vi "UHR-Fleezers Control (host) - Lorentz v3.vi"() -> ()   [LabVIEW 2014] (continued)
  in  "Retract Pump 3":bool
  in  "Stop Flow":bool
  in  "Start Flow":bool
  in  "Flush Sample":bool
  in  "Volume (uL)":dbl=100.0
  in  "Flush rate (uL/m)":dbl=100.0
  in  "Flow rate (uL/h)":dbl=100.0
  in  "Clear Volume":bool caption="Clear Infused Volume"
  in  "Flush Pump 3":bool
  in  "Volume (uL) P3":dbl=150.0 caption="Volume (uL)"
  in  "Flush rate (uL/m) P3":dbl=100.0 caption="Rate (uL/m)"
  out "Flushing P1":bool caption="Flushing"
  in  "Volume (uL) P1":dbl=100.0 caption="Volume (uL)"
  in  "Flush rate (uL/m) P1":dbl=100.0 caption="Rate (uL/m)"
  in  "Normal Flow Rate (ul/h) P1":dbl=600.0 caption="Normal Flow Rate (ul/h)"
  in  "Flush Pump 1":bool
  in  "Clear Volume P3":bool caption="Clear Infused Volume"
  in  "Clear Volume P1":bool caption="Clear Infused Volume"
  in  "Display On P1":bool caption="Display On"
  in  "All Pump Parameters":T10={"Pump 1"={"Diameter (mm)"=4.61, "Units"=4.0, "Volume"=100.0, "Rate"=25.0}, "Pump 2"={"Diameter (mm)"=4.61, "Units"=3.0, "Volume"=0.0, "Rate"=0.0}, "Pump 3"={"Diameter (mm)"=4.61, "Units"=4.0, "Volume"=100.0, "Rate"=800.0}}
  in  "Total Volume\nFlushed (uL)":dbl
  in  "Inject Pump 2":bool caption="Inject Pump 2\n(Flush Center)"
  in  "Flush Center Ch Rate (ul/m)":dbl=100.0
  in  "Flush Center Ch Volume (uL)":dbl=15.0
  in  "Pump pause delay (ms)":u32
  in  "Pump write delay (ms)":dbl=300.0
  in  "Ch 3 Inject Rate (ul/h)":dbl=800.0
  in  "Ch 3 Inject Volume (uL)":dbl=100.0
  in  "Ch 1 Inject Volume (uL)":dbl=100.0
  in  "Ch 1 Inject Rate (ul/h)":dbl=25.0
  out "Pump 1 cont disp":string="Right: DNA beads "
  out "Pump 3 cont disp":string="Left: ADig beads"
  in  "Read Harvard":bool
  out "read buffer":string
  out "Serial Settings:Number of Bytes at Serial Port":u32
  in  "write buffer":string
  in  "Tab Control 2":T11(tab)=enum."Feedback on Trap Position"
  in  "Update all trap values":bool
  out "Total Counts (ticks)":u16=600
  in  "Trap ON/OFF X or Y Amp?":bool=TRUE
  in  "Oscillate Set 1":bool
  in  "Trap 1 ON":bool
  in  "Number Interlace Sets":u8=3 min=1 max=3
  in  "DIO count 3 (ticks)":u16=200
  in  "DIO count 2 (ticks)":u16=200
  in  "DIO count 1 (ticks)":u16=200
  in  "BD 2 Amplitude 3 (%)":dbl min=0.0 max=45.0 step=1.0
  in  "BD 2 Amplitude 2 (%)":dbl min=0.0 max=45.0 step=1.0
  in  "BD 2 Amplitude 1 (%)":dbl min=0.0 max=45.0 step=1.0
  in  "BD 1 Amplitude 3 (%)":dbl min=0.0 max=50.0 step=1.0
  in  "BD 1 Amplitude 2 (%)":dbl=30.0 min=0.0 max=50.0 step=1.0
  in  "BD 1 Amplitude 1 (%)":dbl=30.0 min=0.0 max=50.0 step=1.0
  in  "BD 2 Frequency 3 (MHz)":dbl=26.0 min=0.0 max=40.0 step=0.1 format="%#_6p"
  in  "BD 1 Frequency 3 (MHz)":dbl=70.0 min=60.0 max=90.0 step=1.0 format="%#_6p"
  in  "BD 2 Frequency 2 (MHz)":dbl=26.0 min=0.0 max=40.0 step=0.1 format="%#_6p"
  in  "BD 2 Frequency 1 (MHz)":dbl=26.0 min=0.0 max=40.0 step=0.1 format="%#_6p"
  in  "Not-Interlacing Set":enum32{"Set 1", "Set 2", "Set 3"}(radio)
  in  "Interlace":bool=TRUE
  in  "Trap 2 ON":bool
  in  "Trap 3 ON":bool
  in  "Scan axis 2":bool=TRUE
  in  "Osc. amp. (MHz)":dbl=2.0
  out "Coords":T12
  in  "Manipulation Scaling":cluster{"Horizontal":dbl, "Vertical":dbl}={"Horizontal"=0.075, "Vertical"=0.01}
  in  "Freq or Amp switch first":bool=TRUE
  in  "Swap F1 and F2":bool
  in  "Freq switch delay":u16
  in  "Amp switch delay":u16=7
  in  "BD 1 Delay (ticks)":u8
  in  "BD 2 Delay (Ticks)":u8
  in  "Next trap write delay (ticks)":u8
  in  "XY phase ext loop method":bool
  in  "Amp switch delay 2":u8=5
  in  "BD 2 Delay (Ticks) 2":u8
  in  "BD 1 Delay (ticks) 2":u8
  in  "MCL Step Increment (V_int)":dbl=3.0
  out "Time to Finish All (min)":dbl=0.1665 format="%#_2p"
  in  "Scan Speed (nm/s)":dbl=100.0
  in  "Scan Range (nm)":dbl=500.0
  in  "Step Size (nm)":dbl=1.0
  in  "MCL/AOM Scale Tweak":dbl=1.0
  in  "MCL Step Position Ratio":dbl=0.5
  in  "Move MCL Also?":bool=TRUE
  out "Final sep (nm)":dbl=1398.1532329495126
  out "Initial sep (nm)":dbl=1035.0
  out "Save index":dbl=31.0
  out "Final delta (MHz)":dbl=17.952465308532624
  out "Initial delta (MHz)":dbl=15.0
  out "Final freq. (MHz)":dbl=72.04753469146738
  out "Initial freq. (MHz)":dbl=75.0
  in  "Saved AOD Raster Scan Parameter Sets":T13(array[cluster])=[{"Scan Range AOD (nm) 2"=500.0, "Step Size AOD (nm) 2"=1.0, "Scan Speed AOD (nm/s) 2"=100.0, "Number of scans (AOD) 2"=1, "Label"="offset curve"}, {"Scan Range AOD (nm) 2"=450.0, "Step Size AOD (nm) 2"=1.0, "Scan Speed AOD (nm/s) 2"=100.0, "Number of scans (AOD) 2"=1, "Label"="hp raster check"}, {"Scan Range AOD (nm) 2"=6.8, "Step Size AOD (nm) 2"=0.34, "Scan Speed AOD (nm/s) 2"=0.34, "Number of scans (AOD) 2"=1, "Label"="3.4 kbp - 1 bp steps"}, {"Scan Range AOD (nm) 2"=215.0, "Step Size AOD (nm) 2"=1.0, "Scan Speed AOD (nm/s) 2"=100.0, "Number of scans (AOD) 2"=3, "Label"="dt14 1 14 MHz start"}, {"Scan Range AOD (nm) 2"=450.0, "Step Size AOD (nm) 2"=1.0, "Scan Speed AOD (nm/s) 2"=100.0, "Number of scans (AOD) 2"=1, "Label"="dt14 2 small beads"}, {"Scan Range AOD (nm) 2"=300.0, "Step Size AOD (nm) 2"=1.0, "Scan Speed AOD (nm/s) 2"=100.0, "Number of scans (AOD) 2"=1, "Label"="Oligo"}]
  in  "Load parameters":bool
  out "Scan Range (MHz)":dbl=-2.952465308532625
  in  "Restart DMA? (AOD)":bool=TRUE caption="Restart DMA?"
  out "Incr. int (AOD)":i64=-5635885308
  out "Time/Scan (s) (AOD)":dbl=4.995 format="%#_2p"
  out "Data points/scans":dbl=666000.0
  out "Data points/scan (f/b)":dbl=666000.0
  in  "Save scans":bool=TRUE
  out "AOD Scan I":u64 caption="Scan I"
  in  "Continuous AOD Scanning":bool caption="Continuous Scanning"
  in  "Abort AOD Scan":bool caption="Abort Scan"
  in  "Scan BD":bool=TRUE
  out "Cycles/step (AOD)":u64=666 format="%.3p"
  in  "Number of F/B Scans (AOD)":u16=1 min=1
  out "Scan steps (AOD)":u64=500
  out "Scan Increment (MHz)":dbl=-0.005916764145355961
  out "AOD Scanning":bool caption="Scanning"
  in  "Start AOD Scan":bool caption="Start Scan"
  out "N sets should be saved":dbl=33.3
  out "Progress 2":u16(slide) caption="Progress" scale=0.0..100.0
  in  "Abort save 2":bool caption="Abort save"
  in  "Trap 1 Bead Size (nm)":dbl=810.0
  in  "Trap 2 Bead Size (nm)":dbl=810.0
  out "MCL Count":dbl=541100.8636738182
  in  "Feedback Auto-Off threshold":dbl=9.5
  in  "Trap intensity output range":cluster{"Normal High":i16, "Normal Low":i16}={"Normal High"=3000, "Normal Low"=0}
  in  "All FB On/Off":bool
  in  "AI2 to Setpoint":cluster{"Set 1":bool, "Set 2":bool}
  out "AI2 (V)":cluster{"Set 1":dbl, "Set 2":dbl}={"Set 1"=0.034180730613116855, "Set 2"=0.03936887722403638}
  in  "Reset Feedback":cluster{"Set 1":bool, "Set 2":bool}
  in  "Trap Intensity PID Gains":T14={"proportional gain (Kc)"=10, "integral gain (Kc*Ts/Ti)"=5, "derivative gain (Kc*Td/Ts)"=0}
  in  "Feedback On/Off":cluster{"Set 1":bool, "Set 2":bool}={"Set 1"=TRUE, "Set 2"=TRUE}
  out "Actual Setpoint":fxp<+/-,16,1> format="%.16g"
  in  "Dynamic Force FB (ronen)":bool=TRUE
  in  "Remove Unwinding Offset":bool
  in  "Set Reading to\nSetpoint":bool
  out "Trap X (AI1)":T15={"Trap 1"=-0.25, "Trap 2"=-0.26470947265625}
  in  "Trap Pos FB SP":fxp<+/-,16,1>=0.14581298828125 caption="Setpoint"
  in  "Trap Pos. FB ON":bool
  in  "Reset Trap Pos. FB":bool
  in  "Tab Control 8":T16(tab)
  in  "Red Laser ON/OFF":bool
  in  "Green Laser ON/OFF":bool
  in  "Offset SP2 from SP1":bool
  in  "Use SP 2":bool
  in  "Trap Pos FB Int Count":u16=100
  in  "Trap Pos. FB Gains":T17={"proportional gain (Kc)"=20.0, "integral gain (Kc*Ts/Ti)"=3.0, "derivative gain (Kc*Td/Ts)"=0.0} {"proportional gain (Kc)" format="%.11g"; "integral gain (Kc*Ts/Ti)" format="%.11g"; "derivative gain (Kc*Td/Ts)" format="%.11g"}
  in  "Trap Pos FB SP 2":fxp<+/-,16,1>=-0.10723876953125 caption="Setpoint 2"
  in  "SP2 Offset":fxp<+/-,16,1>=0.100006103515625
  in  "Blue Laser ON/OFF":bool
  in  "Negate Diff?":bool=TRUE
  in  "Differential FB?":bool=TRUE
  in  "Trap Pos. FB Offset Factor":i64
  in  "Trap Pos FB Negate Action":bool=TRUE
  in  "Trap Pos. FB Mult Factor":i64=8388608
  in  "Trap Pos. AI1 X Pre-scale":u16
  in  "Trap Pos. FB Range":T18={"output high"=0.999969482421875, "output low"=-1.0}
  out "Trap Pos FB Int Signal":fxp<+/-,24,9>=13.80865478515625 format="%.18g"
  out "Trap Pos FB Int-Norm Signal":fxp<+/-,16,1>=0.138092041015625 format="%.16g"
  in  "Set SP Using...":bool
  in  "Trap Pos FB Monitor\nT1 or T2":bool
  out "Trap X AI1 (DMA)":T19={"Set 1"=0.999969482421875, "Set 2"=0.999969482421875}
  in  "N El. to Ave.":dbl=10000.0
  out "Trap Pos FB Action":i64
  in  "Target Force (pN)":dbl
  in  "Read Setpoint Correction File":bool
  out "Offset corrected setpoint":fxp<+/-,17,2>
  in  "Real time Offset file correction for setpoint":bool
  out "Offset file step size":dbl
  out "B factor":dbl
  out "Setpoint offset\ncorrection values":dbl[](array[numeric])
  in  "Offset Values":T20={"Trap 1X offset"=array[500 elements], "Trap 2X offset"=array[500 elements]}
  in  "Auto read offset correction":bool=TRUE
  in  "Setpoint Correction Offset File":path=path "C:/Users/Darwin/Desktop/New LabView codes/Thorlabs Motor Codes/Coordinates.txt"
  in  "Dynamic offset\nupdate":bool=TRUE
  in  "Semi Passive Mode":bool
  in  "Jump Force (pN)":dbl
  out "Action (%)":dbl(knob) scale=-100.0..100.0
  in  "Trap Pos. FB Out Scale 2^n":u8=23 caption="Action Scale Factor"
  in  "Remove Action Offset":bool
  in  "factor":dbl
  in  "Tab Control 3":enum32{"Timing", "MCL Scan", "Analog Out"}(tab)
  in  "Initial Phase Adjustment (APD 3 Gate)":i16=80
  in  "Phase Adj. (APD 3 Gate)":i16=20
  in  "+ phase (APD 3 Gate)":bool
  in  "- phase (APD 3 Gate)":bool
  out "APD 2 Gate Late Counter":u8
  out "APD 2 Gate Relative Phase":i16
  in  "Phase Adj. (APD 2 Gate)":i16=1
  in  "Initial Phase Adjustment (APD 2 Gate)":i16=46
  out "APD 1 Gate Late Counter":u8
  in  "- phase (APD 1 Gate)":bool
  in  "+ phase (APD 1 Gate)":bool
  out "APD 1 Gate Relative Phase":i16
  in  "Phase Adj. (APD 1 Gate)":i16=1
  in  "Initial Phase Adjustment (APD 1 Gate)":i16=46
  in  "Save APD Data\nwith Trap Data":bool=TRUE
  out "APD FIFO Elements Remaining":u32=27
  in  "- phase (APD Acq)":bool
  in  "+ phase (APD Acq)":bool
  out "APD Acq Late Counter":u8
  out "APD Acq Relative Phase":i16
  in  "Phase Adj. (APD Acq)":i16=20
  in  "Initial Phase Adjustment (APD Acq)":i16
  in  "Invert APD Gate":bool caption="Invert Gate"
  in  "APD Gate OFF Count":u16=450 caption="Gate OFF Count"
  in  "APD Gate ON Count":u16=150 caption="Gate ON Count"
  in  "APD Gate":enum32{"ON", "OFF", "Interlace"}(radio)=enum."Interlace"
  in  "APD Integration Time (s)":dbl=0.001 caption="Integration Time (s)"
  out "APD Acq Rate (Hz)":dbl=1000.0 caption="Rate (Hz)"
  out "APD Samples/FIFO Acq.":dbl=300.0 caption="Single APD Samples/DMA read"
  out "APD Elements/DMA read":u32=900 caption="All APD Elements/DMA read"
  out "APD Int. Count":u32=40000 format="%.0p"
  in  "+ phase (APD 2 Gate)":bool
  in  "- phase (APD 2 Gate)":bool
  out "APD 3 Gate Late Counter":u8
  out "APD 3 Gate Relative Phase":i16
  out "Number of APDs":u8=3
  in  "Tab Control 5":enum32{"PSD X", "PSD Y", "Other Data Channel"}(tab)
  out "Data map":dbl[][](graph)=[[0.0020383459834110306, 0.0021350803123355933, 0.0022191934211016435, 0.002172709335641655, 0.0030093457648665066, 0.0008064630959880428, 0.0011952292377593252, 0.0026117951080785384, 0.002980212917685829, 0.0017616363498501268, 0.0007388200103561212, 0.001266963900663998, 0.0031927799404533326, 0.002190405042740349, 0.0026020736646468236, 0.002974136249935713, 0.001461473465206213, 0.003565643999009485, 0.0015847870982200036, 0.003126615846359522], [0.0034200981542269818, 0.0010833753907796846, 0.0012214103556302818, 0.0027694408518858515, 0.0023316690006384296, 0.001329750317566862, 0.001045693262943954, 0.0021720396082300195, 0.001057873580644015, 0.0012976270906201368, 0.001844606655106978, 0.0008205636444796576, 0.001884577380298444, 0.0019196100745981653, 0.0035471368506539, 0.0031556116311431803, 0.002772466187518385, 0.003653785229295115, 0.002019577933736527, 0.0026504844733722527], [0.0030435813885914074, 0.003256718331524491, 0.0038435058562425618, 0.001714303315186402, 0.0014131085861415985, 0.0022167116057860313, 0.0018737404243801253, 0.002736979723281846, 0.002203546259039437, 0.0024605540336159045, 0.0015051402523450742, 0.003146798523852864, 0.0022815797146292895, 0.002111235755881686, 0.0031654425893324757, 0.002557286364900697, 0.004405082793797005, 0.0010477533146118889, 0.0018161429228461359, 0.0023148016235006075], [0.002426202849770899, 0.00214256818229328, 0.0034574176134417036, 0.0016245760704472491, 0.0005877313911590428, 0.0024556120116356423, 0.002048585577756134, 0.0018431183520849189, 0.002605734074335316, 0.0017261393853231803, 0.003386039204425333, 0.004260309341867168, 0.0020088395853146376, 0.0024749735875895774, 0.0038215359185463926, 0.0038561467656780587, 0.0020335914257109686, 0.0034785905991928387, 0.0010447838457435703, 0.002604469230421975], [0.0027610691801678686, 0.0029497163131015, 0.0018631508846317152, 0.0019336553047368745, 0.0018312106554342566, 0.0023242068832306836, 0.002396188474980885, 0.002469229592984283, 0.0026677345025492034, 0.0006888790442214515, 0.0019646316328468232, 0.002889551559325103, 0.0024532902964001157, 0.0037818198698241403, 0.002453014197798367, 0.001677016667051827, 0.00302243146165097, 0.0035079968525989183, 0.001958715397227927, 0.003889753098770019], [0.0019422629933325722, 0.0020245151655642925, 0.0015294404751296108, 0.002377583381857813, 0.00161816165776031, 0.000909198116950994, 0.0009075601158313835, 0.0007852171459145706, 0.002228369050598287, 0.0017957689271441645, 0.0011329512328001044, 0.003696230536361944, 0.0027459580307565607, 0.0029594301236012706, 0.0006688170374662072, 0.0023408649049991327, 0.0016154707114121455, 0.0023803968102867924, 0.002207892355047336, 0.002041823353384595], [0.002580440042494945, 0.0022038990649187063, 0.001825805808532021, 0.0017569152930165235, 0.0009898623776115867, 0.002275088649138507, 0.002062169590424864, 0.0005732619451390764, 0.0017308059912430783, 8.933904418400413e-05, 0.0034664628265942913, 0.0028367322638233, 0.0027338494061878867, 0.0037263447117727843, 0.0021997810423537325, 0.003711974166142597, 0.0014771574889931092, 0.0026974988865210367, 0.0027277196692180638, 0.0012765523464854645], [0.002542892311300867, 0.0008387089032983175, 0.0030138051171712805, 0.003855301027336247, 0.0016829395678975134, 0.002327072656777088, 0.0009982286417911973, 0.0014321492145865828, 0.001438368452037204, 0.0018569911695083935, 0.0027217027168985027, 0.0021217440749765485, 0.003997963656267112, 0.001971981481555941, 0.0017950210143396887, 0.0010097906298637738, 0.00269639345065812, 0.0025788239015413447, 0.001985096736536165, 0.00256823316196465], [0.002452298012347215, 0.004392241371176987, 0.0029418361261960993, 0.0024743183397701613, 0.002955614368886482, 0.0012628433287600396, 0.001995570557543791, 0.001841477301731307, 0.0006336584124621782, 0.00038412286187525447, 0.0025754077988013662, 0.003292424542843238, 0.0015884693390730777, 0.0031019967098903107, 0.0012842469220684582, 0.001156701042555189, 0.0019300124803650425, 0.000711833278059485, 0.0025656081840076577, 0.004268434682684796], [0.001291795290455433, 0.002372601738370458, 0.0032183156412125533, 0.0019681766647448905, 0.0037109784546057742, 0.0004291013611950428, 0.0033561663417750473, 0.0015764446752648375, 0.002698558566157524, 0.0015347459346405003, 0.002371931057879887, 0.0017792764974927102, 0.0035202804947955407, 0.0020499903086146597, 0.001205444862530389, 0.0015567818655175657, 0.002647172601612931, 0.0029692488277462434, 0.002515404097249619, 0.002184946088483228], [0.002821327135155408, 0.0023260942250949578, 0.0010912555816772424, 0.0016922959213519825, 0.0027698017187326816, 0.0028569950530006926, 0.0034644518517753997, 0.0016718590844534238, 0.002218951390281129, 0.0038769309546352066, 0.0019126071068609964, 0.0024699377004211804, 0.0014770212736486157, 0.0023162084609381697, 0.0017055477554195554, 0.0016368643290591224, 0.003203999676251886, 0.0032026307826201104, 0.0017932544220486436, 0.002270477268187531], [0.0022278787163343894, 0.0027496469904524337, 0.003625985961023809, 0.004153226104011641, 0.0024166228698149737, 0.0026737177680310805, 0.0019844607789808997, 0.001239111338718075, 0.0016948540928536408, 0.004005193075967077, 0.000630961805097272, 0.0020857235483909497, 0.002248391411474813, 0.0025483315899778513, -0.00014289269800604444, 0.0013990991209830745, 0.002173222163707994, 0.0034697000160164738, 0.002010257683945241, 0.003481043985686529], [0.0018852656320276734, 0.0015715368380061585, 0.0019437671829601755, 0.002470975354509278, 0.0024487910797092428, 0.0007322022696453588, 0.0015475009764890752, 0.0017921866327059758, 0.003058459886432621, 0.0017764067983640703, 0.0025000139148490196, 0.0009623442611020518, 0.0018569165732802914, 0.003310838721775616, 0.00025071352576413444, 0.0036691347962582426, 0.002403046381925506, 0.004055721651469297, 0.002285952907609213, 0.0030062679778400502], [0.0024994380659973843, 0.0026197462346229062, 0.0017527989664171077, 0.0014375842896685127, 0.0033490362530976267, 0.0027052287063586847, 6.381847016474479e-05, 0.0011272327680753905, 0.003454975387457779, 0.004620127122907865, 0.0021178429445671146, 0.004539862151248757, 0.002029684806888378, 0.0013671243967539456, 0.003118446743148983, 0.0010709513970555225, 0.0019090166550763074, 0.002155844648949404, 0.004106378336132433, 0.0010766929367924097], [0.002854938319315421, 0.0038921928444872822, 0.0019246852509770592, 0.001956082424171971, 0.00249396489250124, 0.0024337273809226364, 0.0010765238019800384, 0.002941500719693421, 0.0030759660483101006, 0.0016202953746738819, 0.0017239866140603627, 0.002438327547432977, 0.002786814289877852, 0.002350374795189492, 0.0014284651785432274, 0.0024175263736445143, 0.0017989840672716986, 0.00010277744000073804, 0.0015758938162554312, 0.0015914808231177855], [0.0023379764512881855, 0.0019152406361689915, 0.0023721211744209382, 0.0028072318841611175, 0.00045998972816663626, 0.0019525984204332083, 0.001965702699358644, 0.0032523064679092764, 0.000928270862367026, 0.0025551238347956457, 0.0027235426100884804, 0.0006003323047511277, 0.0024452031525158107, 0.003200615692319165, 0.0031679408338207383, 0.001713752296656085, 0.0029069566496737467, 0.0017760622106257355, 0.0032846637736200987, 0.0014145046584398283], [0.0017413311095229888, 0.002850684453478228, 0.004119312336274303, 0.001376098161794153, 0.0028391954791758406, 0.0023504256794032296, 0.001939098372782241, 0.0009962144963960734, 0.0017508511614465492, 0.0010266285265010658, 0.00317450379791817, 0.002092576486750102, 0.003523745928434037, 0.003362704188893568, 0.0022223282833307503, 0.003285433624934814, 0.0021443498633667525, 0.0006378287745106628, 0.0009042965230192737, 0.004364189912157604], [0.0025684771943308964, 0.003595940600289024, 0.0015386127114892655, 0.002970017638684016, 0.000731008903710616, 0.0015627389249673368, 0.00268734680621615, 0.00033321301039761556, 0.002657761688265375, 0.0018452193301245214, 0.0019648865080461276, 0.00321862929090469, 0.002422721362346656, 0.0036160768033011536, 0.0023323715302130984, 0.0016526314538286777, 0.0033099223028642, 0.0014149263891099, 0.00254445644786201, 0.002714841511848489], [0.00302323496353701, 0.0016076200915618212, 0.001298400361326538, 0.0018074432822074325, 0.0026357010223677386, 0.002293142925429444, 0.001403310979000166, 0.002185113177831846, 0.002789454480226071, 0.0017208525559712065, 0.0017792513529249357, 0.0019822099798379907, 0.0028293142834817267, 0.002262865370925418, 0.001290800627866991, 0.0023298166748236485, 0.0013506602320411689, 0.002143358706259156, 0.0035532369528369174, 0.0017335871199569027], [0.0025192336907101567, 0.0023420394966944366, 0.0018803373952631193, 0.0019133833353522055, 0.0012596720449505453, 0.002147060132875675, 0.0006990538240453468, 0.0021223766921043765, 0.0033568805410328644, 0.0019950947049262504, 0.0021300391805659505, 0.001813624441258409, 0.0011352622065457982, 0.002742817450067307, 0.002825619560905981, 0.0028865080849197105, 0.003418778555540925, 0.0015302210369144652, 0.004455456383213908, 0.0013599469983302684], [-0.0004438837985084353, 0.0028183355707480946, 0.0028130708775573115, 0.0030206214884492544, 3.0807351233010224e-06, 0.00100356141409364, 0.003239142551743778, 0.0028015305417013713, 0.0016360555337629936, 0.0021630034342628546, 0.002737139846047398, 0.0036584890379432007, 0.002471730052534626, 0.0023361339599424456, 0.0029788411839639624, 0.0014442602794432905, 0.0023810759191331154, 0.0012413151489925564, 0.0019023668482100798, 0.002640107429201507], [0.001554782428247715, 0.002954419634687952, 0.0028951557424149637, 0.003310458814954959, 0.002365836700244099, 0.0030819547506098647, 0.0022846439376502706, 0.00043219002702368965, 0.003015949202071104, 0.002476214118282937, 0.0012666534517914985, 0.003753630460609294, 0.0019762301625312097, 0.0024128905675427107, 0.0024715495496260395, 0.0012053557199650255, 0.0030770984437811398, 0.001260030580666012, 0.002103542906975703, 0.003243844033696315], [0.002047169886274074, 0.003135570533130444, 0.003659218345652883, 0.003351918820368115, 0.002638669639842362, 0.0032054173808839705, 0.002728466251491257, 0.002422436287272547, 0.0027550251027393968, 0.0011484124718350213, 0.0024811181138690744, 0.000633754661919369, 0.004103389272200948, 0.002413442590560708, 0.0010161905814301843, 0.0006117013741451642, 0.00043229932014902874, 0.0026398449564406256, 0.002421923707756009, 0.0037337823125722382], [0.003223733537026557, 0.0018388836414569803, 0.0009593646694003638, 0.002150504738108695, 0.002240376826733987, 0.002819775892773071, 0.0023671589694118722, 0.000575767662750824, 0.002985254604568729, 0.0016894905303978737, 0.0022470149983889803, 0.0003279829367159081, 0.0036647064650229947, 0.0034208513812910607, 0.001372326074939035, 0.0012329776908317572, 0.0021677603380249777, 0.002634189260273172, 0.0028446181528041406, 0.00213113583206634], [0.0019954076065657263, 0.0037723924706211747, 0.001706529185397683, 0.002364821147683791, 0.002979725244773599, 0.0025437175845808863, 0.0021453554509108016, 0.004057319159369964, 0.003080980549531066, 0.002721994671347667, 0.0023390951175459806, 0.00256423096986864, 0.0028016019632848403, 0.004136674747509183, 0.0013482163844892154, 0.0025822615725757214, 0.0036704638004895884, 0.0027356369424274387, 0.0026386812531819896, 0.004017865052466032], [0.0024523481698112215, 0.001577397825690218, 0.003482073577677887, 0.0013120929321507693, 0.0023779996424196947, 0.0031885279055957677, 0.0030968142000769574, 0.0008079901646664205, 0.002057639245236158, 0.0014454916165466576, 0.0024913028609758626, 0.0037321652111583048, 0.0017568129726518262, 0.002433957686700396, 0.0013519635336044248, 0.0025583649394570035, 0.0028389004443714833, 0.0022371439658448768, 0.0027243471248494314, 0.0029988024916099377], [0.004482728416008117, 0.002106313095020212, 0.0016966090569018176, 0.002396355324914029, 0.0028921242144040655, 0.0015488778727110483, 0.003087584542752191, 0.0015783381053925663, 0.002107198839582597, 0.002028492535057995, 0.002133558230340132, 0.0033792319972435966, 0.0027693102835735124, 0.0018097134809963325, 0.0018729748671947632, 0.002639158100819596, 0.0020228765137224065, 0.0027609921089093853, 0.0018507896888375831, 0.0037945518126489184], [0.0021563482581923206, 0.0032287318120543937, 0.002708679733426596, 0.001050676702211846, 0.0025215820393785435, 0.0028877563801691696, 0.0019552140449292524, 0.0008869258799717261, 0.00135938852287414, 0.0018791457864769595, 0.0023044366557142164, 0.001505864205337834, 0.002869003954012599, 0.002875615556306393, 0.0002350922247605644, 0.001003648267132261, 0.002356427438894899, 0.0023482204070056395, 0.0030151148802336925, 0.0028427289795750045], [0.0038551731030675492, 0.0032190719566552277, 0.0024841888185482774, 0.0021509928606914825, 0.0019762178118407662, 0.0010938081355370294, 0.0013139616940169843, 0.0021720191912326476, 0.0022752909556785724, 0.001220901184309662, 0.0016582026045028472, 0.0024335127088734292, 0.0024787123106594982, 0.0020212943620039874, 0.0016344163085200308, 0.000406346466621824, 0.0029532673665144445, 0.0024979601850372486, 0.0026392577111319635, 0.004397563792842481], [0.0019392152337034533, 0.0025752001941428933, 0.002375394930020305, 0.0028141695664536765, 0.0030603007029344938, 0.0011131838617945628, 0.002016520759374347, 0.0007694648026350759, 0.0015220876353260865, 0.0007363225146947519, 0.000638103757805431, 0.0021367847621378373, 0.0006798563886399791, 0.0030144489262747447, 0.0012521090204634475, 0.0008366649244029356, 0.0025666821561406115, 0.001756081969563725, 0.0032417664621542308, 0.0027129101328840412], [0.004234965435631261, 0.0028807923900716586, 0.003994864856813696, 0.002228016783386847, 0.0020643224474904383, 0.0032080385730002244, 0.0024267095326168985, 0.0017045994219985895, 0.0004388872799201384, 0.0033081602061115307, 0.001876598014475262, 0.002967363816837642, 0.0014745477365160986, 0.0020882770356405143, 0.0013540441866247209, -0.0006440024187520807, 0.0028524616240076846, 0.0014866404270267755, 0.00212329751615424, 0.0033980422597344436], [0.002443103566818908, 0.0028643225076063544, 0.0026559502913978718, 0.0037632868164488202, 0.002284871036146773, 0.0015618259048538988, 0.0017562004198199274, 0.0013422612594893234, 0.0021296203269845397, 0.0025582835925385674, 0.0014546337054565813, 0.0012911088291717825, 0.0016512241182034806, 0.0022875704433646493, 0.003230826380294793, 0.0017297408349598563, 0.0026936683465980803, 0.0034380066316832677, 0.0020340691324621275, 0.0024417322062178165], [-9.989324566289746e-05, 0.002926244866839386, 0.0012902951621840647, 0.0026901742294294408, 0.0007707616757238599, 0.002362816916091356, 0.001011706400022051, 0.0017386970379252784, 0.0020217996444839735, 0.002564324057587132, 7.627346006863279e-05, 0.0002802241821891143, 0.0026582840805945995, 0.004267218692043419, 0.0008375444339060319, 0.001425992926040155, 0.0018555300552344036, 0.0019526652519745082, 0.0035856622760482276, 0.003574377792936731], [0.0022162866870525226, -9.80488992076956e-05, 0.0025575817989724257, 0.0017415298145425548, 0.0027732403933223874, 0.001805105566650088, 0.003135078437970281, 0.00030140619095551545, 0.002650648973281749, 0.0017502683903315023, 0.0010009292556551102, -0.0001580201494951381, 0.002096695649478786, 0.0023734494130614623, 0.001871656497385907, 0.0010147521269191551, 0.0028769559123858206, 0.001535512363638828, 0.0016771158914974686, 0.0036812015349025297], [0.0032911157382341976, 0.0015937673246648396, 0.0022786049298841506, 0.0016435202933210561, -0.000444139543920988, 0.0010322872285660274, 0.0015058197657779827, 0.0015226621305386731, 0.0013670575927993015, 0.001993129770992985, 0.0024129146141866654, -0.000271958439995209, 0.0032173265132192236, 0.001258442789528919, 0.0017013782876058627, 0.002937335820531526, 0.0020141218387929012, 0.00339081594854371, 0.0023237992039019865, 0.0019362936150417998], [0.0010726759952865783, 0.00383807561043779, 0.0038445499562823364, 0.0037327075782894294, 0.0030324176425392917, 0.000939469808843528, 0.0033586682713470056, 0.0007949762712558317, 0.0026842935481138233, 0.0027066995591428656, 0.001000126612503554, 0.0010644965226183879, 0.0012534863266311373, 0.000971090044070356, 0.0020274176610303746, 0.001313872990779878, 0.004415055089640197, 0.0022069739121942404, 0.000147794314328749, 0.003687654343198644], [0.0013238774283048135, 0.0016832656412011497, 0.002987102709259717, 0.0030815330868127306, 0.0029175865629059517, 0.001487872746945953, 0.0026091093679822507, 0.00135137082614052, 0.0011924192830799123, 0.002261800469194393, 0.000771417004330296, 0.0023250295522089758, 0.0016879132492112036, 0.0019726696926899378, 0.001788107104334166, 0.003862482787623552, 0.0024858537507722227, 0.00385855737054356, 0.0015301935270155484, 0.0031097752029073805], [0.0022271538965262065, 0.002149103591341216, 0.0008579581902112741, 0.0030474920826782247, 0.0032464784941930586, 0.002202404463612722, 0.0028610862175354876, 0.00119149906196459, 0.001159386660592406, 0.0010568905868378246, 0.0016045775757651311, 0.002078856957174876, 0.0031696706950223794, 0.0015400561930039819, 0.0018392034125027834, 0.0019016707318218183, 0.0025078250875444456, 0.0021647130900559666, 0.0006667868013903893, 0.002689612407972146], [0.003174915343868663, 0.0017082274160115402, 0.0004799123732484494, 0.002356906409014597, 0.002454123557174727, 0.0019283029529754366, 0.0005167238834184597, 0.0010390784903798918, 0.0022056908793985446, 0.0027450940851695103, 0.0015664249441001616, 0.0025970210907853447, 0.0031492312654002328, 0.0023489673010236925, 0.0016732664571149716, 0.0023468000185280606, 0.0006955608188309671, 0.0009160564453459453, 0.002208430013051778, 0.0010033313743313265], [0.002771809170291859, 0.0013473649729025135, 0.0020308167485843616, 0.0033787301181636546, 0.00265669183861397, 0.002015256758420677, 0.0021247098216520435, 0.001977968519838654, 0.0034117189837875477, 0.0017658010805061703, 0.0025104575542475244, 0.002180588571631346, 0.0027725271015961524, 0.0036683916030291934, 0.00346879977795831, 0.0016237785338239006, 0.0013883707480767996, 0.0030502992866057047, 0.0031019819698129046, 0.0016354795807633777]]
  in  "Channel":i32=4
  in  "Abort MCL Scan":bool
  out "MCL Scan I":u64
  out "MCL Scanning":bool
  in  "Start MCL Scan":bool
  out "wait to reset values":bool
  in  "Tab Control 4":enum32{"Scan Settings", "MCL FPGA Loop Timing"}(tab)
  out "Total Time (s)":dbl=4.8
  in  "Scan lines (y)":u64=20
  in  "Fast Scan Dir":bool=TRUE
  in  "2D or 1D Scan":bool=TRUE
  out "Initial X":dbl=1.3285729544969032
  out "Initial Y":dbl=4.00431745353557
  out "Time/f+b scan (s) (MCL)":dbl=0.24 caption="Time/scan (s)"
  in  "Number of scans (MCL)":u64=1 caption="Scans"
  in  "Scan steps (MCL)":u64=40 caption="Scan steps (x)"
  in  "N APD Samp/step":dbl=3.0
  in  "Scan Range (V)\n(of steps)":dbl=7.0
  in  "Restart DMA? (MCL)":bool=TRUE caption="Restart DMA?"
  in  "Continuous MCL Scanning":bool caption="Cont. Scanning"
  in  "Center Scan":bool=TRUE
  in  "Save Data (MCL)":bool=TRUE caption="Save Data"
  out "Actual Incr. int (MCL)":i16=588 caption="Incr. int"
  out "Desired incr (int)":dbl=588.125641025641
  out "Desired Scan Incr (V)":dbl=0.1794871794871795
  out "N sets should be saved (MCL)":dbl=16.0 caption="N sets should be saved"
  out "Data points/scans (MCL)":dbl=4800.0 caption="Data points/scans"
  out "Data points/scan (f+b)":dbl=240.0 caption="points/scan (f+b)"
  out "Cycles/step (MCL)":u64=200 caption="Cycles/step" format="%.0p"
  out "Actual MCL Inc (V)":dbl=0.1794488357188635
  in  "Phase adjust (MCL)":i16 caption="Phase adjust"
  out "Relative Phase (MCL)":i16 caption="Relative Phase"
  in  "Initial Phase Adj. (MCL)":i16 caption="Initial Phase Adj."
  in  "Update Count (MCL)":u32=600
  in  "+ phase (MCL)":bool
  in  "- phase (MCL)":bool
  out "MCL Late Counter":u8
  in  "APD AO Scale Factor":i16=1 min=1
  in  "Fluorescent excitation laser controls":T21(tab)
  in  "Interlace OFF count":u16=450 min=1 step=1
  in  "Interlace ON count":u16=150 min=1 step=1
  in  "Duty Frequency (ON 1/N cycles)":u16=1
  in  "Invert laser interlacing":bool
  out "Fluorescence laser intensities plot":cluster{dbl, dbl, dbl}(graph)
  in  "Green FB On/Off":bool
  in  "Red FB On/Off":bool
  in  "Blue FB On/Off":bool
  in  "Red Intensity % (FB OFF)":dbl=20.0 min=0.0 max=100.0 step=1.0
  in  "Blue Intensity % (FB OFF)":dbl=87.0 min=0.0 max=100.0 step=1.0
  out "Green laser intensity (V)":dbl
  in  "Initial Phase Adjustment (Green FB)":i16=-30
  in  "Phase adj. (Green FB)":i16=10
  out "Green AI Count":u16=600
  in  "- phase (Green FB)":bool
  in  "+ phase (Green FB)":bool
  out "Relative phase (Green FB)":i16
  out "GI Late Counter 2":u8
  in  "Phase adj. (GI) 2":i16=1
  out "GI relative phase 2":i16
  in  "+ phase (GI) 2":bool
  in  "Initial Phase Adjustment (GI) 2":i16=-274
  in  "- phase (GI) 2":bool
  in  "Green FB Gains":T14={"proportional gain (Kc)"=10, "integral gain (Kc*Ts/Ti)"=5, "derivative gain (Kc*Td/Ts)"=0}
  in  "Green int current ON count adj":u32=150
  in  "- phase (GI)":bool
  in  "Initial Phase Adjustment (GI)":i16=-28
  in  "+ phase (GI)":bool
  out "GI relative phase":i16
  in  "Phase adj. (GI)":i16=1
  out "GI Late Counter":u8
  out "Green AI Late Counter":u8
  out "MCL Scan":cluster{"Begin (V)":dbl, dbl, dbl[]}(graph)
  out "MCL Scan 2":cluster{"Begin (V)":dbl, dbl, dbl[]}(graph)
  out "Red laser intensity (V)":dbl
  out "Red AI Count":u16=600
  in  "Initial Phase Adjustment (RI)":i16=25
  out "RI Late Counter":u8
